vi "Get Property.vi"(10 "Ctl Ref":refnum<vi>, 11 "UIP In":refnum<class "TipStripUIP.lvclass">) -> (0 "Error Out":errorcluster, 3 "UIP Out":refnum<class "TipStripUIP.lvclass">)   [LabVIEW 2020, in "UIM.lvlib" / "TipStripUIP.lvclass"]
doc: "Modify this method to implement functionality for extracting the property from VI Server Control to be stored inside UIP."
uses:
  TipStripUIP.lvclass
  TipStripUIP.lvclass/TipStripUIP.ctl
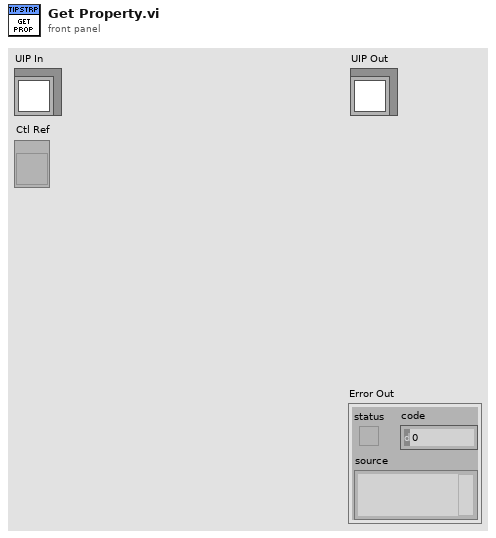
[diagram p1: front panel]
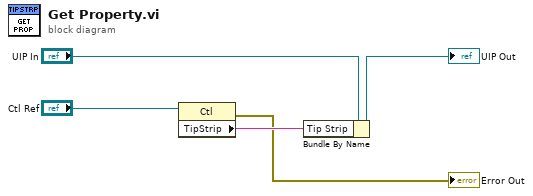
[diagram p0: block diagram]
diagram:
  n1 = property class="Ctl"(reference="Ctl Ref") -> (error out=→"Error Out":errorcluster, "TipStrip"=w3:string)  [unwired: 1 in, 1 out]
  n2 = Bundle By Name(cluster="UIP In", "Tip Strip"=w3) -> (→"UIP Out":refnum<class "TipStripUIP.lvclass">)
